vi "Projet peletier.vi"() -> ()   [LabVIEW 2022 SP3]
uses:
  <vilib>/MakerHub/LINX/LMH-LINX.lvlib
  <vilib>/MakerHub/LINX/Public/Peripherals/Digital/Digital Write N Chans.vi
  <vilib>/vision/driver/NI_Vision_Acquisition_Software.lvlib
  <vilib>/vision/NI_Vision_Development_Module.lvlib
  <vilib>/MakerHub/LINX/Public/Utilities/Open Serial.vi
  <vilib>/userDefined/High Color/IMAQdx.ctl
panel:
  in  "Images/s":sgl(knob)=1.0 min=1 max=10 step=1 scale=0.0..10.0 scale format="%#.6g"
  out "température":dbl
  in  "Zone du texte à lire :":T1 {"Rotation" min=-90.0 max=90.0 step=1.0 format="%.2f"; "Left" scale=0.0..1024.0; "Right" scale=0.0..1024.0}
  out "Refroidissement en cours":string
  out "Chauffage en cours":string
  in  "OK Button":bool
  out "Selection":string
  in  "Arduino":refnum<visa-resource-name>="COM3"
  out "Image":T2(plugin-control)
  out "Temps d'inertie (s)":dbl caption="Elapsed Time (s)" format="%#_4g"
  in  "Caméra":T3="cam1"
  out "Evolution de la température en fonction du temps":cluster{"Value":dbl[], "Value":dbl[]}(graph)
  in  "Veuillez entrer la température voulue":dbl
  out "X":dbl[](array[numeric])
  out "Y":dbl[](array[numeric])
  out "enregistrement de la température":dbl
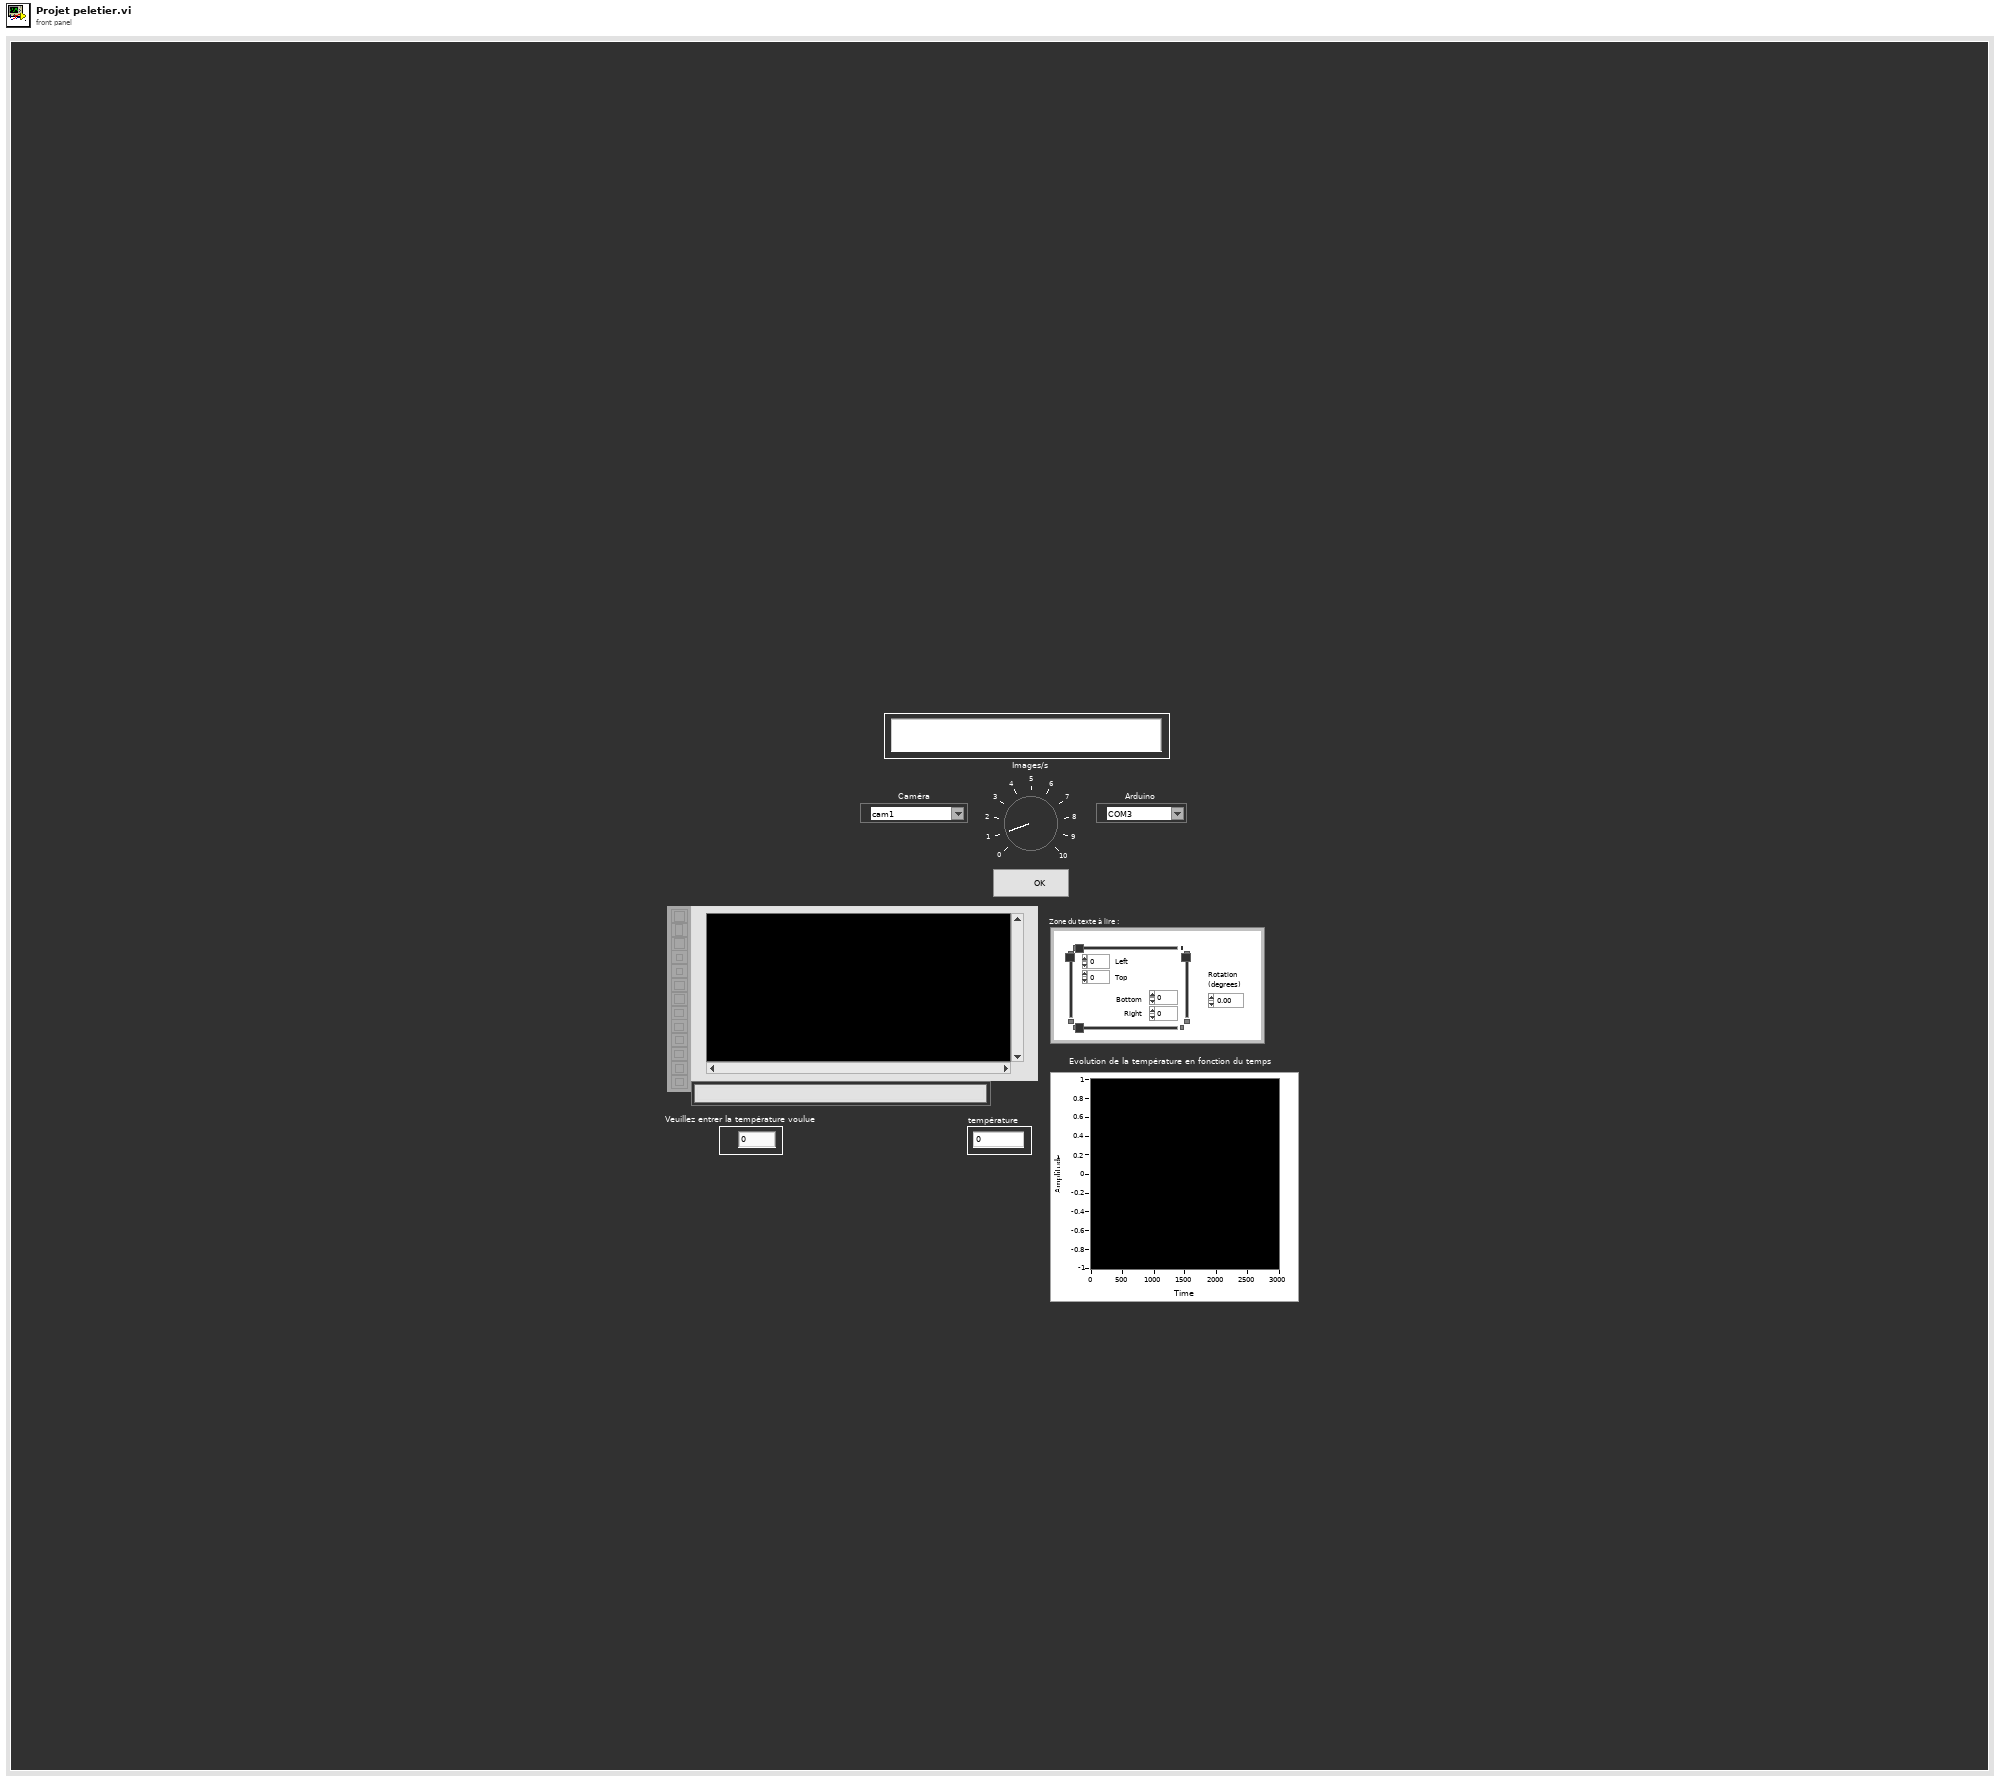
[diagram p1: front panel]
types:
  T1 = typedef "IMAQ Rectangle" = cluster{"Left":i32, "Top":i32, "Right":i32, "Bottom":i32, "Rotation":dbl}
  T2 = typedef "IMAQ Image.ctl" = refnum<image>
  T3 = typedef "IMAQdx.ctl" = refnum<k21>
  T4 = typedef "LMH-LINX.lvlib/LINX Ref.ctl" = cluster{"IO":T5, "Interface":T6, "LINX Device Config":T7}
  T5 = typedef "LMH-LINX.lvlib/Platform.ctl" = enum16{"Remote", "Local"}
  T6 = typedef "LMH-LINX.lvlib/Interface.ctl" = enum16{"Serial", "TCP"}
  T7 = typedef "LMH-LINX.lvlib/Device.lvlib/LINX Device Config.ctl" = cluster{"Interface":T6, "COM Port":refnum<visa-resource-name>, "TCP Configuration":T8, "Device Family":u8, "Device ID":u8, "Device Name":string, "TCP Ref":refnum<k5>, "Channels":T9}
  T8 = typedef "LMH-LINX.lvlib/Device.lvlib/TCP Config.ctl" = cluster{"IP Address":string, "Port":u16}
  T9 = typedef "LMH-LINX.lvlib/Channels.ctl" = cluster{"DI":u8[], "DO":u8[], "AI":u8[], "AO":u8[], "PWM":u8[], "QE":u8[], "UART":u8[], "I2C 2":u8[], "SPI":u8[], "CAN":u8[], "Servo":u8[], "AI Ref (V)":dbl, "AI Resolution (Bits)":u8, "AO Ref (V)":dbl, "AO Resolution (Bits)":u8}
  T10 = typedef "IMAQ OCR Session.ctl" = refnum<k1>
  T11 = typedef "ROI Descriptor" = cluster{"Global Rectangle":i32[], "Contours":cluster{"ID":enum32{"External", "Internal"}, "Type":u32, "Coordinates":i32[]}[]}
  T12 = typedef "IMAQ Point" = cluster{"X":sgl, "Y":sgl}
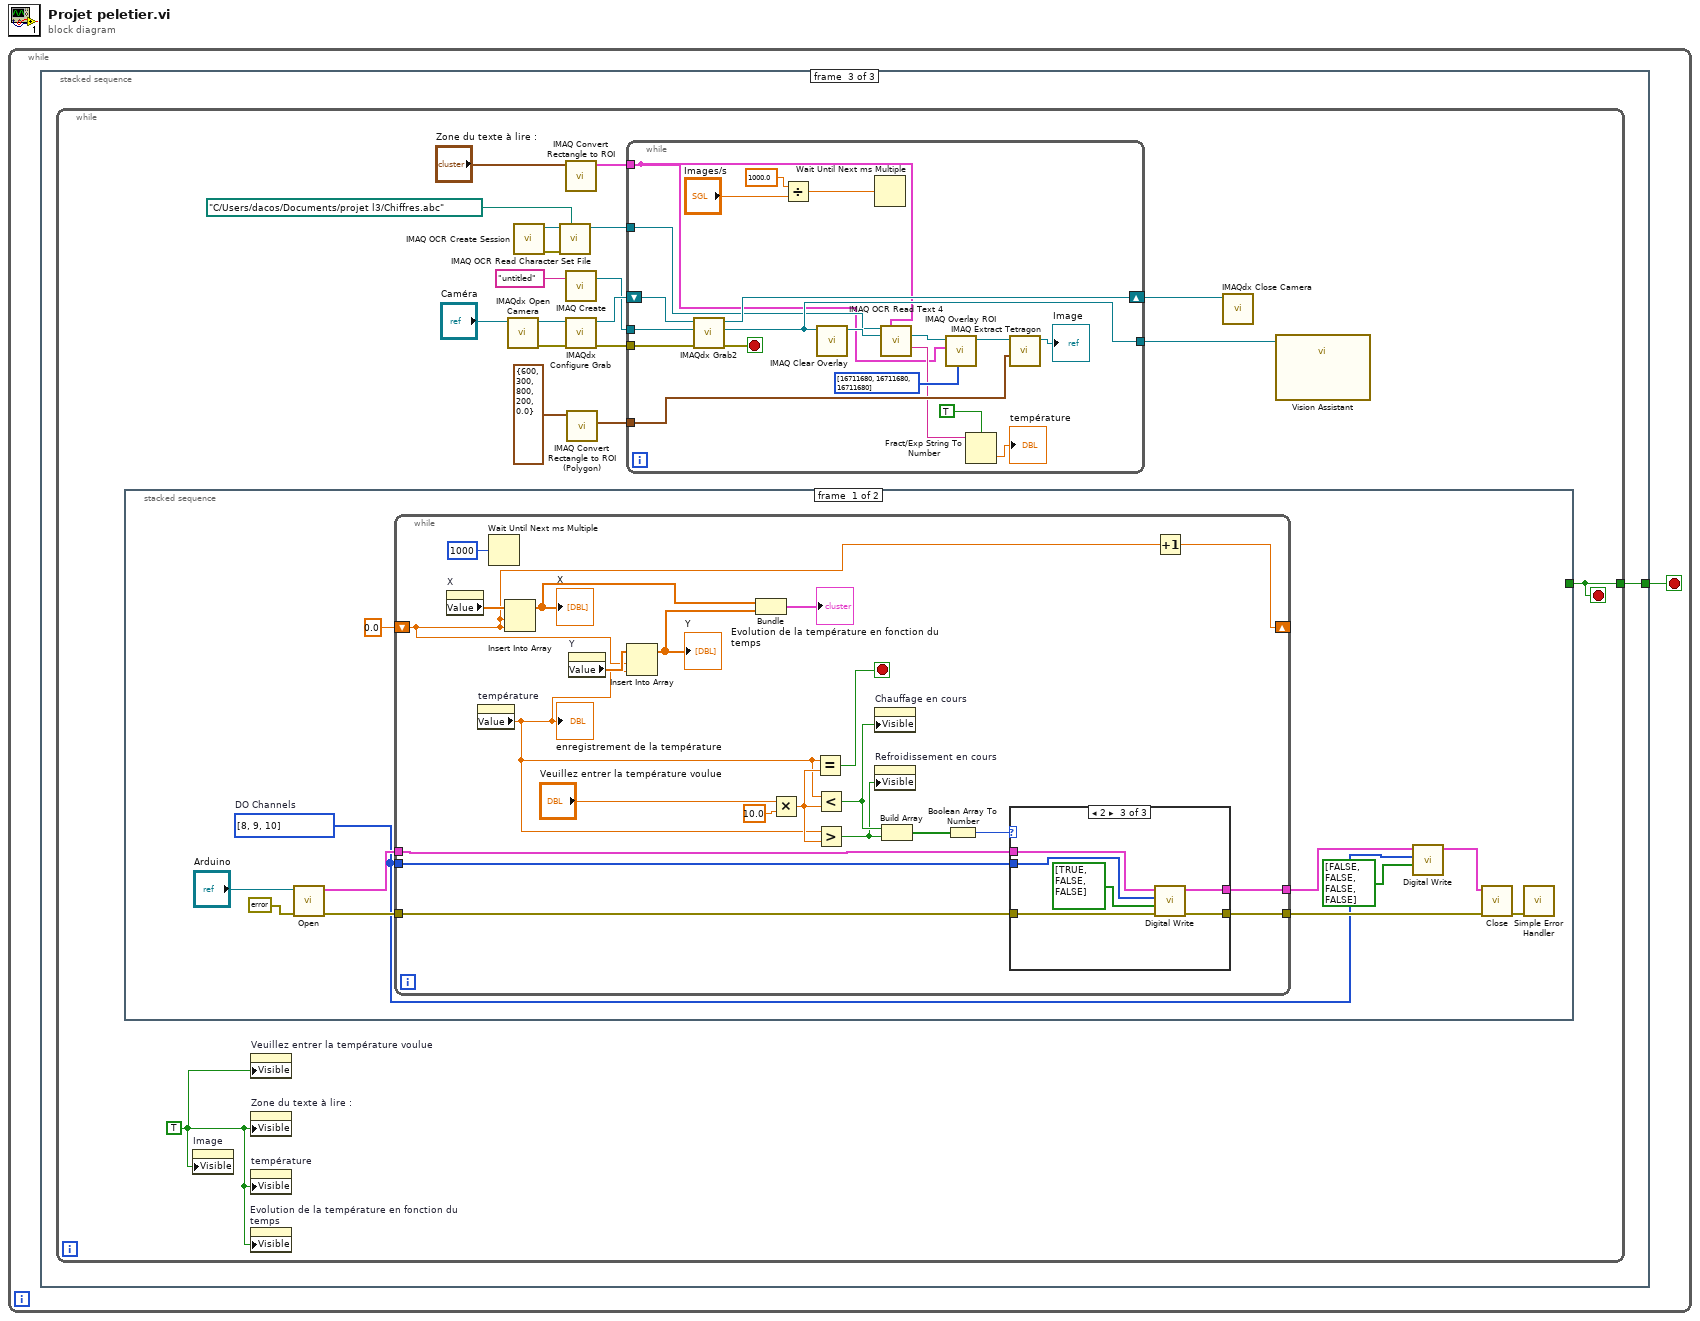
[diagram p0: block diagram]
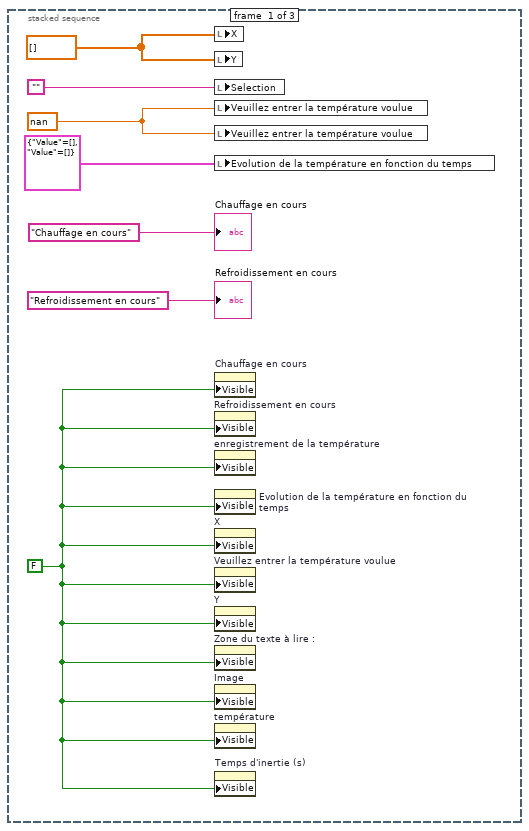
[diagram p2: hidden frame]
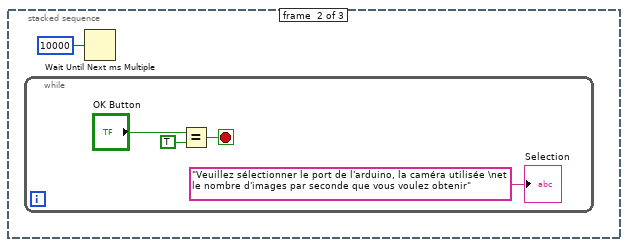
[diagram p3: hidden frame]
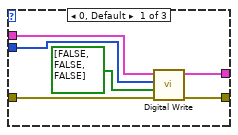
[diagram p4: hidden frame]
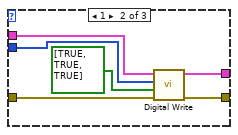
[diagram p5: hidden frame]
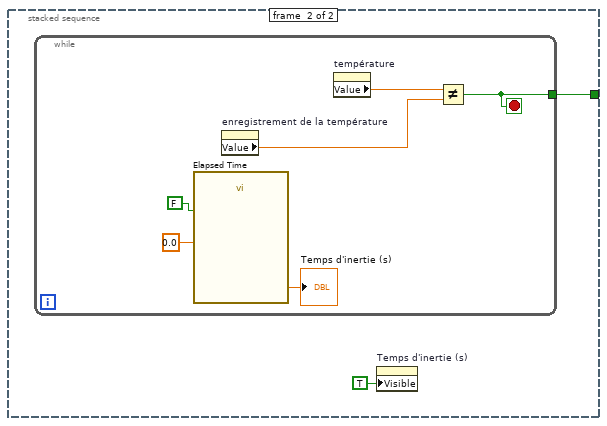
[diagram p6: hidden frame]
diagram:
  n1 = while {
    stop <- w1 stop-if-true
    n2 = stacked-sequence {
      tunnel: [_ _ w14] -> w1
      frame #0 {
        w3 = nan
        w2 = FALSE
        w6 = dbl[] [] ("Y")
        n3 = local write "X"(w6) -> ()
        n4 = local write "Y"(w6) -> ()
        n5 = local write "Selection"("") -> ()
        n6 = local write "Veuillez entrer la température voulue"(w3) -> ()
        n7 = local write "Veuillez entrer la température voulue"(w3) -> ()
        n8 = local write "Evolution de la température en fonction du temps"(cluster{"Value":dbl[], "Value":dbl[]} {"Value"=[], "Value"=[]} ("Evolution de la température \nen fonction du temps")) -> ()
        n9 = property on="Chauffage en cours" class="Str"("Visible"=w2) -> ()  [unwired: 2 in, 2 out]
        n10 = property on="Refroidissement en cours" class="Str"("Visible"=w2) -> ()  [unwired: 2 in, 2 out]
        n11 = property on="enregistrement de la température" class="DigNum (strict)"("Visible"=w2) -> ()  [unwired: 2 in, 2 out]
        n12 = property on="Evolution de la température en fonction du temps" class="XYGraph (strict)"("Visible"=w2) -> ()  [unwired: 2 in, 2 out]
        n13 = property on="X" class="Arr (strict)"("Visible"=w2) -> ()  [unwired: 2 in, 2 out]
        n14 = property on="Veuillez entrer la température voulue" class="DigNum (strict)"("Visible"=w2) -> ()  [unwired: 2 in, 2 out]
        n15 = property on="Y" class="Arr (strict)"("Visible"=w2) -> ()  [unwired: 2 in, 2 out]
        n16 = property on="Zone du texte à lire :" class="Clust (strict)"("Visible"=w2) -> ()  [unwired: 2 in, 2 out]
        n17 = property on="Image" class="ImageControl"("Visible"=w2) -> ()  [unwired: 2 in, 2 out]
        n18 = property on="température" class="DigNum (strict)"("Visible"=w2) -> ()  [unwired: 2 in, 2 out]
        n19 = property on="Temps d'inertie (s)" class="DigNum (strict)"("Visible"=w2) -> ()  [unwired: 2 in, 2 out]
        "Refroidissement en cours" <- "Refroidissement en cours" ("Refroidissement en cours")
        "Chauffage en cours" <- "Chauffage en cours" ("Chauffage en cours")
      }
      frame #1 {
        n20 = while {
          stop <- w10 stop-if-true
          n21 = Equal?(x="OK Button", y=TRUE) -> (x = y?=w10:bool)
          "Selection" <- "Veuillez sélectionner le port de l'arduino, la caméra utilisée \net le nombre d'images par seconde que vous voulez obtenir"
        }
        n22 = Wait Until Next ms Multiple(millisecond multiple=u32 10000) -> ()  [unwired: 1 out]
      }
      frame #2 {
        n23 = while {
          tunnel: [w16] -> w14
          stop <- w16 stop-if-true
          w15 = TRUE
          n24 = stacked-sequence {
            tunnel: [_ w106] -> w16
            frame #0 {
              w56 = u8[] [8, 9, 10]  # DO Channels
              n25 = call-poly <vilib>:"Open.vi"("Error In"=errorcluster {"status"=FALSE, "code"=0, "source"=""}, "Serial Port"="Arduino") -> ("Error Out"=w63:errorcluster, "LINX Resource"=w64:T4)  [unwired: 7 in, 1 out]
              n26 = while {
                tunnel: w64 -> [w83]
                tunnel: w63 -> [w79]
                tunnel: [w82] -> w58
                tunnel: [w81] -> w61
                tunnel: w56 -> [w80]
                shift-right: [w76] -> _
                shift-left: 0.0 ("x") -> [w74]
                stop <- w68 stop-if-true
                n27 = property on="X" class="Arr (strict)"() -> ("Value"=w77:dbl[])  [unwired: 2 in, 2 out]
                n28 = property on="température" class="DigNum (strict)"() -> ("Value"=w65:dbl)  [unwired: 2 in, 2 out]
                "enregistrement de la température" <- w65
                n29 = Wait Until Next ms Multiple(millisecond multiple=u32 1000 ("milliseconds to wait")) -> ()  [unwired: 1 out]
                n30 = Insert Into Array(array=w77, index=w74, new element=w74) -> (w73:dbl[])
                "X" <- w73
                n31 = property on="Y" class="Arr (strict)"() -> ("Value"=w78:dbl[])  [unwired: 2 in, 2 out]
                n32 = Insert Into Array(array=w78, index=w74, new element=w65) -> (w72:dbl[])
                "Y" <- w72
                n33 = Bundle("Value"=w73, "Value"=w72) -> (→"Evolution de la température en fonction du temps":cluster{"Value":dbl[], "Value":dbl[]})  [unwired: 1 in]
                n34 = Multiply(x="Veuillez entrer la température voulue", y=10.0) -> (x*y=w71:dbl)
                n35 = Equal?(x=w65, y=w71) -> (x = y?=w68:bool)
                n36 = Less?(x=w65, y=w71) -> (x < y?=w67:bool)
                n37 = Greater?(x=w65, y=w71) -> (0:w66:bool)
                n38 = property on="Chauffage en cours" class="Str"("Visible"=w67) -> ()  [unwired: 2 in, 2 out]
                n39 = property on="Refroidissement en cours" class="Str"("Visible"=w66) -> ()  [unwired: 2 in, 2 out]
                n40 = Build Array(w67, w66) -> (w85:bool[])
                n41 = Boolean Array To Number(Boolean array=w85) -> (number=w84:u32)
                n42 = case shown="2" w84 {
                  tunnel: w83 -> [w89 w98 w104]
                  tunnel: [w90 w97 w103] -> w82
                  tunnel: [w91 w96 w101] -> w81
                  tunnel: w80 -> [w87 w95 w102]
                  tunnel: w79 -> [w92 w93 w99]
                  frame 0, Default {
                    n43 = call-poly <vilib>:"Digital Write.vi"("Error In"=w92, "Values"=bool[] [FALSE, FALSE, FALSE], "DO Channels"=w87, "LINX Resource"=w89) -> ("Error Out"=w91:errorcluster, "LINX Resource"=w90:T4)  [unwired: 6 in]
                  }
                  frame 1 {
                    n44 = call-poly <vilib>:"Digital Write.vi"("Error In"=w93, "Values"=bool[] [TRUE, TRUE, TRUE], "DO Channels"=w95, "LINX Resource"=w98) -> ("Error Out"=w96:errorcluster, "LINX Resource"=w97:T4)  [unwired: 6 in]
                  }
                  frame 2 {
                    n45 = call-poly <vilib>:"Digital Write.vi"("Error In"=w99, "Values"=bool[] [TRUE, FALSE, FALSE], "DO Channels"=w102, "LINX Resource"=w104) -> ("Error Out"=w101:errorcluster, "LINX Resource"=w103:T4)  [unwired: 6 in]
                  }
                }
                n46 = Increment(x=w74) -> (x+1=w76:dbl)
              }
              n47 = call-poly <vilib>:"Digital Write.vi"("Values"=bool[] [FALSE, FALSE, FALSE, FALSE], "DO Channels"=w56, "LINX Resource"=w58) -> ("LINX Resource"=w57:T4)  [unwired: 7 in, 1 out]
              n48 = call <vilib>:"Close.vi"("Error In"=w61, "LINX Resource"=w57) -> ("Error Out"=w60:errorcluster)  [unwired: 9 in]
              n49 = call <vilib>:"Simple Error Handler.vi"("error in (no error)"=w60) -> ()  [unwired: 4 in, 5 out]
            }
            frame #1 {
              n50 = while {
                tunnel: [w107] -> w106
                stop <- w107 stop-if-true
                n51 = call "Elapsed Time"("Auto Reset"=FALSE, "Set Start Time (s)"=0.0) -> ("Elapsed Time (s)"=→"Temps d'inertie (s)":dbl)  [unwired: 10 in, 7 out]
                n52 = property on="enregistrement de la température" class="DigNum (strict)"() -> ("Value"=w109:dbl)  [unwired: 2 in, 2 out]
                n53 = property on="température" class="DigNum (strict)"() -> ("Value"=w108:dbl)  [unwired: 2 in, 2 out]
                n54 = Not Equal?(x=w108, y=w109) -> (x != y?=w107:bool)
              }
              n55 = property on="Temps d'inertie (s)" class="DigNum (strict)"("Visible"=TRUE) -> ()  [unwired: 2 in, 2 out]
            }
          }
          n56 = property on="Image" class="ImageControl"("Visible"=w15) -> ()  [unwired: 2 in, 2 out]
          n57 = property on="Veuillez entrer la température voulue" class="DigNum (strict)"("Visible"=w15) -> ()  [unwired: 2 in, 2 out]
          n58 = property on="Zone du texte à lire :" class="Clust (strict)"("Visible"=w15) -> ()  [unwired: 2 in, 2 out]
          n59 = property on="température" class="DigNum (strict)"("Visible"=w15) -> ()  [unwired: 2 in, 2 out]
          n60 = property on="Evolution de la température en fonction du temps" class="XYGraph (strict)"("Visible"=w15) -> ()  [unwired: 2 in, 2 out]
          n61 = call <vilib>:"IMAQdx Open Camera.vi"("Session In"="Caméra") -> ("error out"=w32:errorcluster, "Session Out"=w33:T3)  [unwired: 9 in]
          n62 = call "IMAQ OCR Create Session"() -> ("error out"=w26:errorcluster, "IMAQ OCR Session"=w27:T10)  [unwired: 10 in]
          n63 = call "IMAQ OCR Read Character Set File"("File Path"=path "C:/Users/dacos/Documents/projet l3/Chiffres.abc", "error in (no error)"=w26, "IMAQ OCR Session"=w27) -> ("IMAQ OCR Session (dup)"=w24:T10)  [unwired: 6 in, 2 out]
          n64 = call "IMAQ Convert Rectangle to ROI"("Rectangle"="Zone du texte à lire :") -> ("ROI Descriptor"=w23:T11)  [unwired: 8 in, 1 out]
          n65 = call "IMAQ Create"("Image Name"="untitled") -> ("New Image"=w17:T2)  [unwired: 4 in, 1 out]
          n66 = call <vilib>:"IMAQdx Configure Grab.vi"("error in"=w32, "Session In"=w33) -> ("error out"=w29:errorcluster, "Session Out"=w31:T3)  [unwired: 8 in]
          n67 = call "IMAQ Convert Rectangle to ROI (Polygon)"("Rectangle"=T1 {"Left"=600, "Top"=300, "Right"=800, "Bottom"=200, "Rotation"=0.0}) -> ("Rectangle Points"=w21:T12[])  [unwired: 7 in, 2 out]
          n68 = while {
            tunnel: w29 -> [w52]
            shift-right: [w51] -> w28
            shift-left: w31 -> [w53]
            tunnel: w24 -> [w44]
            tunnel: w23 -> [w40]
            tunnel: [w45] -> w22
            tunnel: w21 -> [w43]
            tunnel: w17 -> [w37]
            stop <- w50 stop-if-true
            n69 = call <vilib>:"IMAQdx Grab2.vi"("error in"=w52, "Image In"=w37, "Session In"=w53) -> ("error out"=w50:errorcluster, "Image Out"=w45:T2, "Session Out"=w51:T3)  [unwired: 5 in, 1 out]
            n70 = Divide(x=sgl 1000.0, y="Images/s") -> (x/y=w34:sgl)
            n71 = call "IMAQ Clear Overlay"("Image"=w45) -> ("Image Out"=w47:T2)  [unwired: 9 in, 1 out]
            n72 = Wait Until Next ms Multiple(millisecond multiple=w34) -> ()  [unwired: 1 out]
            n73 = call "IMAQ OCR Read Text 4"("IMAQ OCR Session"=w44, "ROI Descriptor"=w40, "Image"=w47) -> ("Image (dup)"=w49:T2, "Read String"=w41:string)  [unwired: 6 in, 5 out]
            n74 = call "IMAQ Overlay ROI"("Colors (Green)"=u32[] [16711680, 16711680, 16711680], "ROI Descriptor"=w40, "Image"=w49) -> ("Image Out"=w42:T2)  [unwired: 7 in, 1 out]
            n75 = Fract/Exp String To Number(use system decimal point (T)=TRUE, string=w41) -> (number=→"température":dbl)  [unwired: 2 in, 1 out]
            n76 = call-poly "IMAQ Extract Tetragon"("Tetragon"=w43, "Image Src"=w42) -> ("Image Dst Out"=→"Image":T2)  [unwired: 8 in, 1 out]
          }
          n77 = call <vilib>:"IMAQdx Close Camera.vi"("Session In"=w28) -> ()  [unwired: 10 in, 1 out]
          n78 = call "Vision Assistant"("Image In"=w22) -> ()  [unwired: 25 in, 2 out]
        }
      }
    }
  }
